vi "firstDemo.vi"() -> ()   [LabVIEW 2021]
panel:
  in  "stop":bool
  out "Waveform Graph":dynamicdata(graph)
  in  "Feq":dbl(knob) scale=0.0..10.0
  in  "Amp":dbl(knob) scale=0.0..10.0
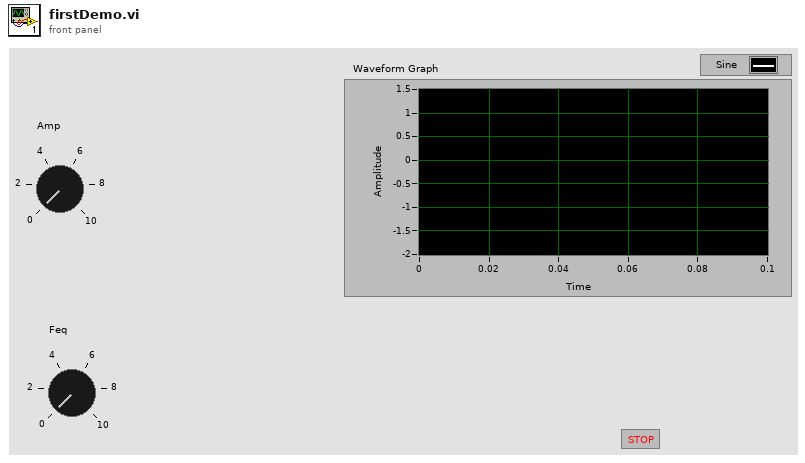
[diagram p1: front panel]
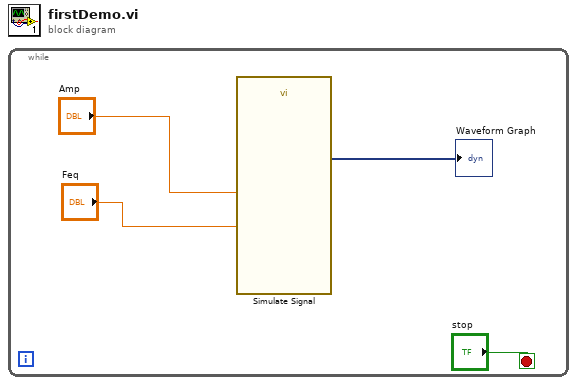
[diagram p0: block diagram]
diagram:
  n1 = while {
    stop <- "stop" stop-if-true
    n2 = call "Simulate Signal"("Frequency"="Feq", "Amplitude"="Amp") -> ("Sine"=→"Waveform Graph":dynamicdata)  [unwired: 12 in, 1 out]
  }
